vi "Ref_Mask.vi"(0 "Mask Ch 1":refnum<vi>, 1 "Mask Ch 2":refnum<vi>, 2 "Mask Ch 3":refnum<vi>, 3 "Mask Ch 4":refnum<vi>, 4 "Mask Ch 5":refnum<vi>, 5 "Mask Ch 6":refnum<vi>, 6 "Mask Ch 7":refnum<vi>, 7 "Mask Ch 8":refnum<vi>, 8 "Mask Ch 9":refnum<vi>, 9 "Mask Ch 10":refnum<vi>, 14 "Init_F":bool=TRUE) -> (18 "Mask Ch 9 out":refnum<vi>, 19 "Mask Ch 10 out":refnum<vi>, 20 "Mask Ch 1 out":refnum<vi>, 21 "Mask Ch 2 out":refnum<vi>, 22 "Mask Ch 3 out":refnum<vi>, 23 "Mask Ch 4 out":refnum<vi>, 24 "Mask Ch 5 out":refnum<vi>, 25 "Mask Ch 6 out":refnum<vi>, 26 "Mask Ch 7 out":refnum<vi>, 27 "Mask Ch 8 out":refnum<vi>)   [LabVIEW 2017]
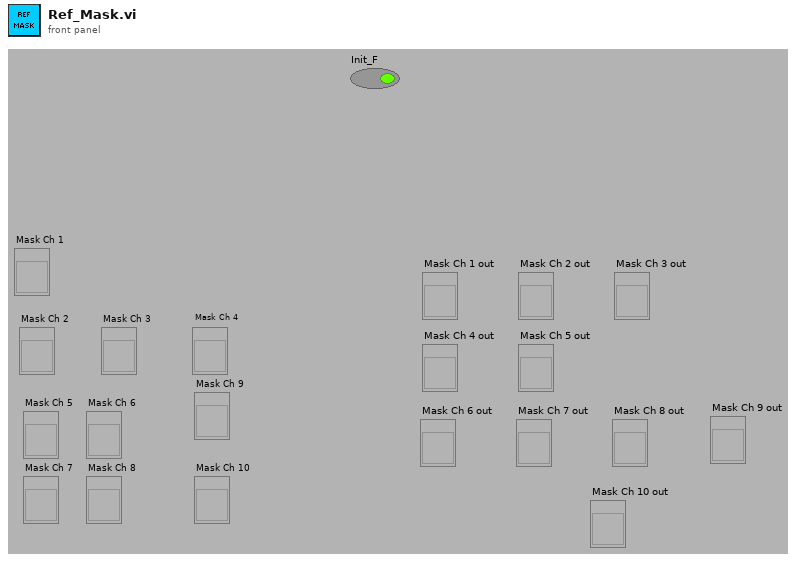
[diagram p1: front panel]
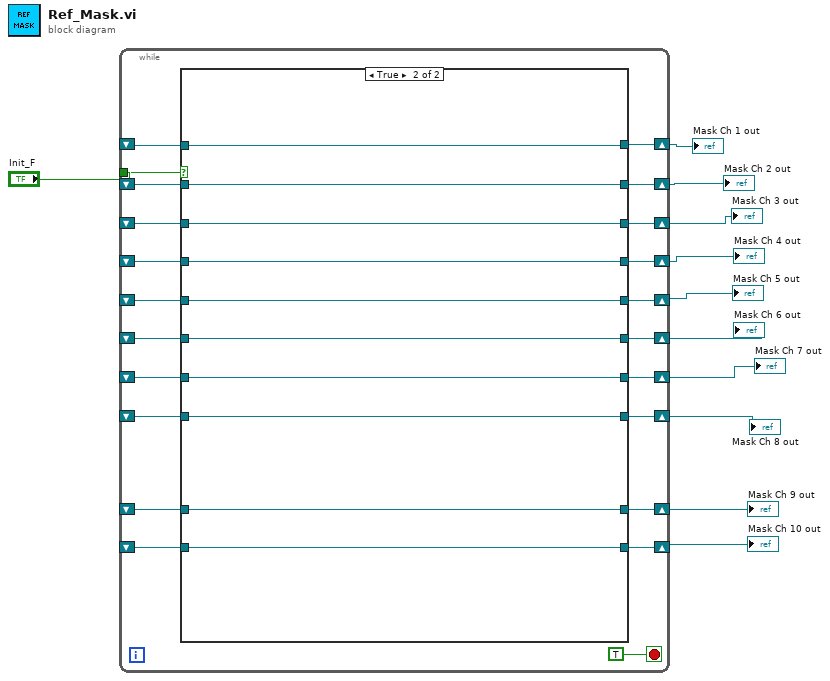
[diagram p0: block diagram]
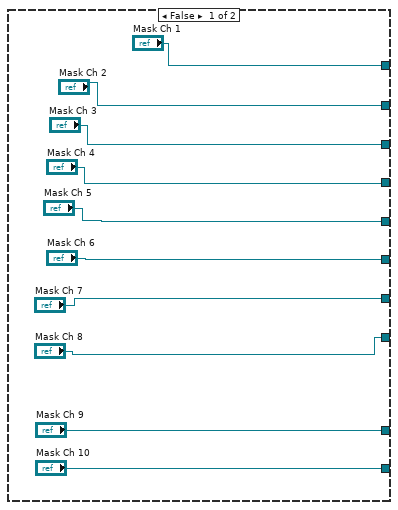
[diagram p2: hidden frame]
diagram:
  n1 = while {
    shift-right: [w32] -> w10
    shift-left: _ -> [w31]
    tunnel: "Init_F" -> [w30]
    shift-right: [w29] -> w9
    shift-left: _ -> [w22]
    shift-right: [w28] -> w8
    shift-left: _ -> [w21]
    shift-right: [w27] -> w7
    shift-left: _ -> [w16]
    shift-right: [w26] -> w6
    shift-left: _ -> [w20]
    shift-right: [w25] -> w5
    shift-left: _ -> [w19]
    shift-right: [w24] -> w4
    shift-left: _ -> [w18]
    shift-right: [w23] -> w3
    shift-left: _ -> [w17]
    shift-right: [w15] -> w2
    shift-left: _ -> [w13]
    shift-right: [w14] -> w1
    shift-left: _ -> [w12]
    stop <- TRUE stop-if-true
    n2 = case shown="True" w30 {
      tunnel: ["Mask Ch 1" w53] -> w32
      tunnel: w31 -> [_ w53]
      tunnel: ["Mask Ch 2" w46] -> w29
      tunnel: ["Mask Ch 3" w47] -> w28
      tunnel: ["Mask Ch 4" w48] -> w27
      tunnel: ["Mask Ch 5" w49] -> w26
      tunnel: ["Mask Ch 6" w50] -> w25
      tunnel: ["Mask Ch 7" w51] -> w24
      tunnel: ["Mask Ch 8" w52] -> w23
      tunnel: w22 -> [_ w46]
      tunnel: w21 -> [_ w47]
      tunnel: w20 -> [_ w49]
      tunnel: w19 -> [_ w50]
      tunnel: w18 -> [_ w51]
      tunnel: w17 -> [_ w52]
      tunnel: w16 -> [_ w48]
      tunnel: ["Mask Ch 9" w45] -> w15
      tunnel: ["Mask Ch 10" w44] -> w14
      tunnel: w13 -> [_ w45]
      tunnel: w12 -> [_ w44]
      frame False {
      }
      frame True {
      }
    }
  }
  "Mask Ch 1 out" <- w10
  "Mask Ch 2 out" <- w9
  "Mask Ch 3 out" <- w8
  "Mask Ch 4 out" <- w7
  "Mask Ch 5 out" <- w6
  "Mask Ch 6 out" <- w5
  "Mask Ch 7 out" <- w4
  "Mask Ch 8 out" <- w3
  "Mask Ch 9 out" <- w2
  "Mask Ch 10 out" <- w1
